vi "Prepare Control.vi"(7 "VolatusAPI":refnum<class "VolatusAPI.lvclass">, 8 "error in (no error)":errorcluster, 11 "ValveControl in":refnum<class "ValueSetControl.lvclass">) -> (0 "error out":errorcluster, 3 "ValveControl out":refnum<class "ValueSetControl.lvclass">)   [LabVIEW 2020, in "VolatusControl.lvlib" / "ValueSetControl.lvclass"]
uses:
  ValueSetControl.lvclass
  Volatus/VolatusAPI/VolatusAPI.lvclass
  ValueSetControl.lvclass/ValueSetControl.ctl
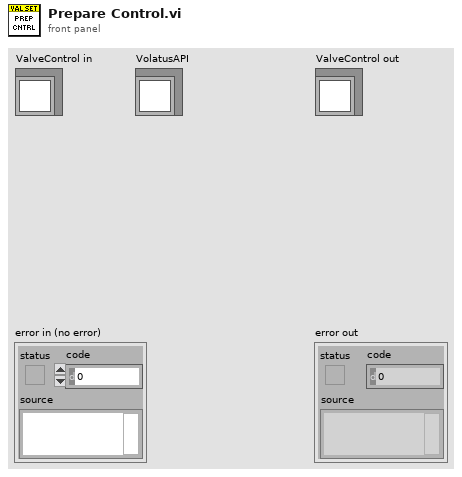
[diagram p1: front panel]
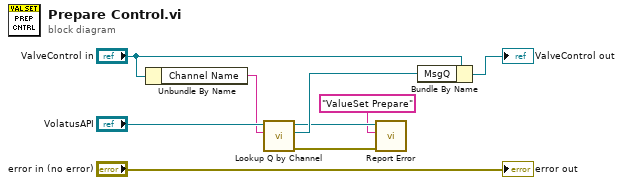
[diagram p0: block diagram]
diagram:
  n1 = Unbundle By Name("ValveControl in") -> ("Channel Name"=w7:string)
  n2 = call "Lookup Q by Channel.vi"("Channel Name"=w7, "VolatusAPI in"="VolatusAPI") -> ("error out"=w2:errorcluster, "MessageQ"=w5:refnum<class "MessageQ.lvclass">, "VolatusAPI out"=w3:refnum<class "VolatusAPI.lvclass">)  [unwired: 7 in]
  n3 = call "Report Error.vi"("error in (no error)"=w2, "Context"="ValueSet Prepare", "VolatusAPI in"=w3) -> ()  [unwired: 7 in, 2 out]
  n4 = Bundle By Name(cluster="ValveControl in", "MsgQ"=w5) -> (→"ValveControl out":refnum<class "ValueSetControl.lvclass">)
  "error out" <- "error in (no error)"
